vi "getAdditionalDataFromXMLNative.vi"(8 "error in (no error)":errorcluster, 10 "eventXML":refnum<k20>, 11 "RfRamp in":refnum<class "RfRamp.lvclass">) -> (0 "error out":errorcluster, 2 "eventXML out":refnum<k20>, 3 "RfRamp out":refnum<class "RfRamp.lvclass">)   [LabVIEW 2009, in "Tools.lvlib" / "Scripting.lvlib" / "RfRamp.lvclass"]
uses:
  RfRamp.lvclass
  <vilib>/xml/Close Reference(Node).vi
  RfRamp.lvclass/RfRamp.ctl
  <vilib>/xml/NI_XML.lvlib
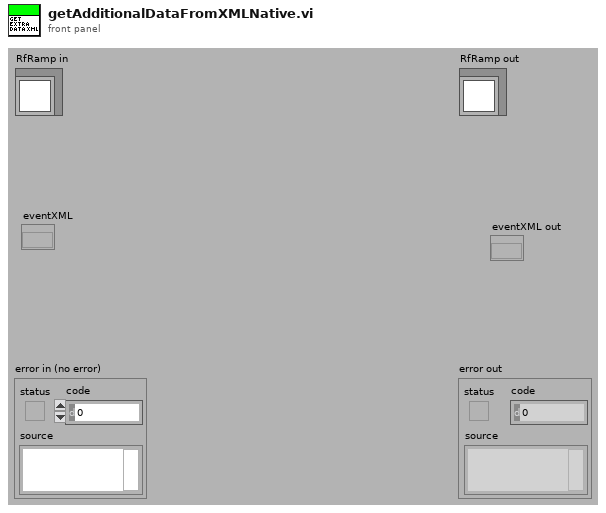
[diagram p1: front panel]
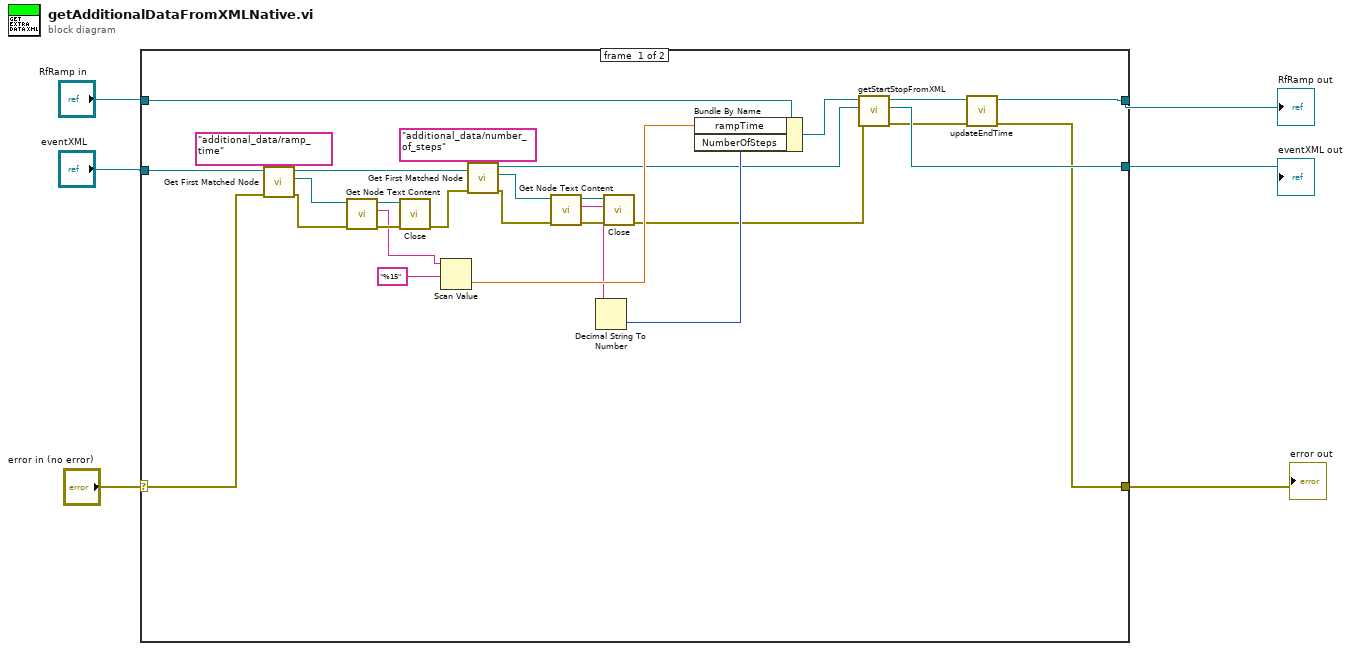
[diagram p0: block diagram]
diagram:
  n1 = case shown="No Error" "error in (no error)" {
    selector: "error in (no error)" -> [w30 w36]
    tunnel: [w7 w36] -> w2
    tunnel: [w8 w37] -> w3
    tunnel: "RfRamp in" -> [w18 w37]
    tunnel: "eventXML" -> [w31 w35]
    tunnel: [w12 w35] -> w1
    frame #0 {
      n2 = call <vilib>:"Get First Matched Node.vi"("error in (no error)"=w30, "XPath expression"="additional_data/ramp_time", "node in"=w31) -> ("error out"=w27:errorcluster, "node result"=w28:refnum<k20>, "node out"=w21:refnum<k20>)  [unwired: 6 in]
      n3 = call <vilib>:"Get Node Text Content.vi"("error in (no error)"=w27, "node in"=w28) -> ("error out"=w32:errorcluster, "node text"=w19:string, "node out"=w33:refnum<k20>)  [unwired: 7 in]
      n4 = call-poly <vilib>:"Close.vi"("error in (no error)"=w32, "node"=w33) -> ("error out"=w20:errorcluster)  [unwired: 7 in]
      n5 = Scan Value(string=w19, format string="%15") -> (value=w17:dbl)  [unwired: 1 in, 1 out]
      n6 = call <vilib>:"Get First Matched Node.vi"("error in (no error)"=w20, "XPath expression"="additional_data/number_of_steps", "node in"=w21) -> ("error out"=w26:errorcluster, "node result"=w25:refnum<k20>, "node out"=w13:refnum<k20>)  [unwired: 6 in]
      n7 = call <vilib>:"Get Node Text Content.vi"("error in (no error)"=w26, "node in"=w25) -> ("error out"=w23:errorcluster, "node text"=w16:string, "node out"=w22:refnum<k20>)  [unwired: 7 in]
      n8 = Decimal String To Number(string=w16) -> (number=w15:i32)  [unwired: 2 in, 1 out]
      n9 = call-poly <vilib>:"Close.vi"("error in (no error)"=w23, "node"=w22) -> ("error out"=w11:errorcluster)  [unwired: 7 in]
      n10 = Bundle By Name(cluster=w18, "rampTime"=w17, "NumberOfSteps"=w15) -> (w14:refnum<class "RfRamp.lvclass">)
      n11 = call "getStartStopFromXML.vi"("error in (no error)"=w11, "eventXML"=w13, "RfRamp in"=w14) -> ("error out"=w9:errorcluster, "eventXML out"=w12:refnum<k20>, "RfRamp out"=w10:refnum<class "RfRamp.lvclass">)  [unwired: 6 in]
      n12 = call-dynamic "updateEndTime.vi"("error in (no error)"=w9, "RfRamp in"=w10) -> ("error out"=w7:errorcluster, "RfRamp out"=w8:refnum<class "RfRamp.lvclass">)  [unwired: 8 in]
    }
    frame #1 {
    }
  }
  "error out" <- w2
  "RfRamp out" <- w3
  "eventXML out" <- w1
